vi "And.vi"(4 "b":bool, 5 "a":bool) -> (1 "out":bool)   [LabVIEW 2014]
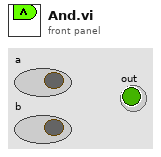
[diagram p1: front panel]
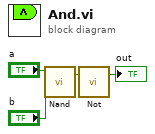
[diagram p0: block diagram]
diagram:
  n1 = call "Nand.vi"("b"="b", "a"="a") -> ("out"=w2:bool)  [unwired: 3 in]
  n2 = call "Not.vi"("in"=w2) -> ("out"=→"out":bool)  [unwired: 2 in]
